vi "Creators Status Created Queues.vi"(11 "eeeee in":refnum<class "eeeee.lvclass">) -> (0 "Created Queue Count":i32, 1 "Created Queue Aliases":string[](array[string]), 2 "Created Queue Exist?":bool, 3 "eeeee out":refnum<class "eeeee.lvclass">)   [LabVIEW 2021, in "Providers.lvlib" / "eeeee.lvlib" / "eeeee.lvclass"]
uses:
  eeeee.lvclass
  eeeee.lvclass/eeeee.ctl
  jettl/Event/Event.lvclass
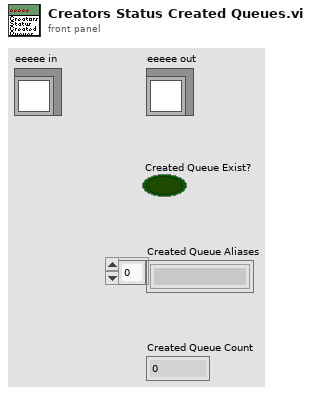
[diagram p1: front panel]
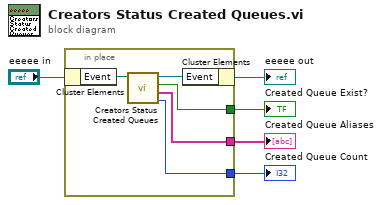
[diagram p0: block diagram]
diagram:
  n1 = in-place {
    in-place-border: [w8] -> w3
    in-place-border: [w7] -> w2
    in-place-border: [w6] -> w1
    n2 = in-place-cluster #1("eeeee in") -> ("Event"=w10:refnum<class "Event.lvclass">)
    n3 = call-dynamic "Creators Status Created Queues.vi"("Event in"=w10) -> ("Created Queue Count"=w6:i32, "Created Queue Aliases"=w7:string[], "Created Queue Exist?"=w8:bool, "Event out"=w9:refnum<class "Event.lvclass">)  [unwired: 7 in]
    n4 = in-place-cluster #1("Event"=w9) -> (→"eeeee out":refnum<class "eeeee.lvclass">)
  }
  "Created Queue Exist?" <- w3
  "Created Queue Aliases" <- w2
  "Created Queue Count" <- w1
